vi "CheckPressure.vi"(8 "error in (no error)":errorcluster, 11 "UI.lvclass":refnum<class "S3.lvclass">) -> (0 "error out":errorcluster, 3 "UI.lvclass 2":refnum<class "S3.lvclass">)   [LabVIEW 2018, in "S3.lvclass"]
uses:
  S3.lvclass
  S3.lvclass/S3.ctl
  Public Controls/ReportHeader.ctl
  GUI2/GUI2.lvclass
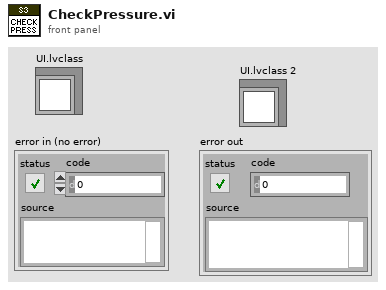
[diagram p1: front panel]
types:
  T1 = typedef "S3.lvclass/ReportHeader.ctl" = string
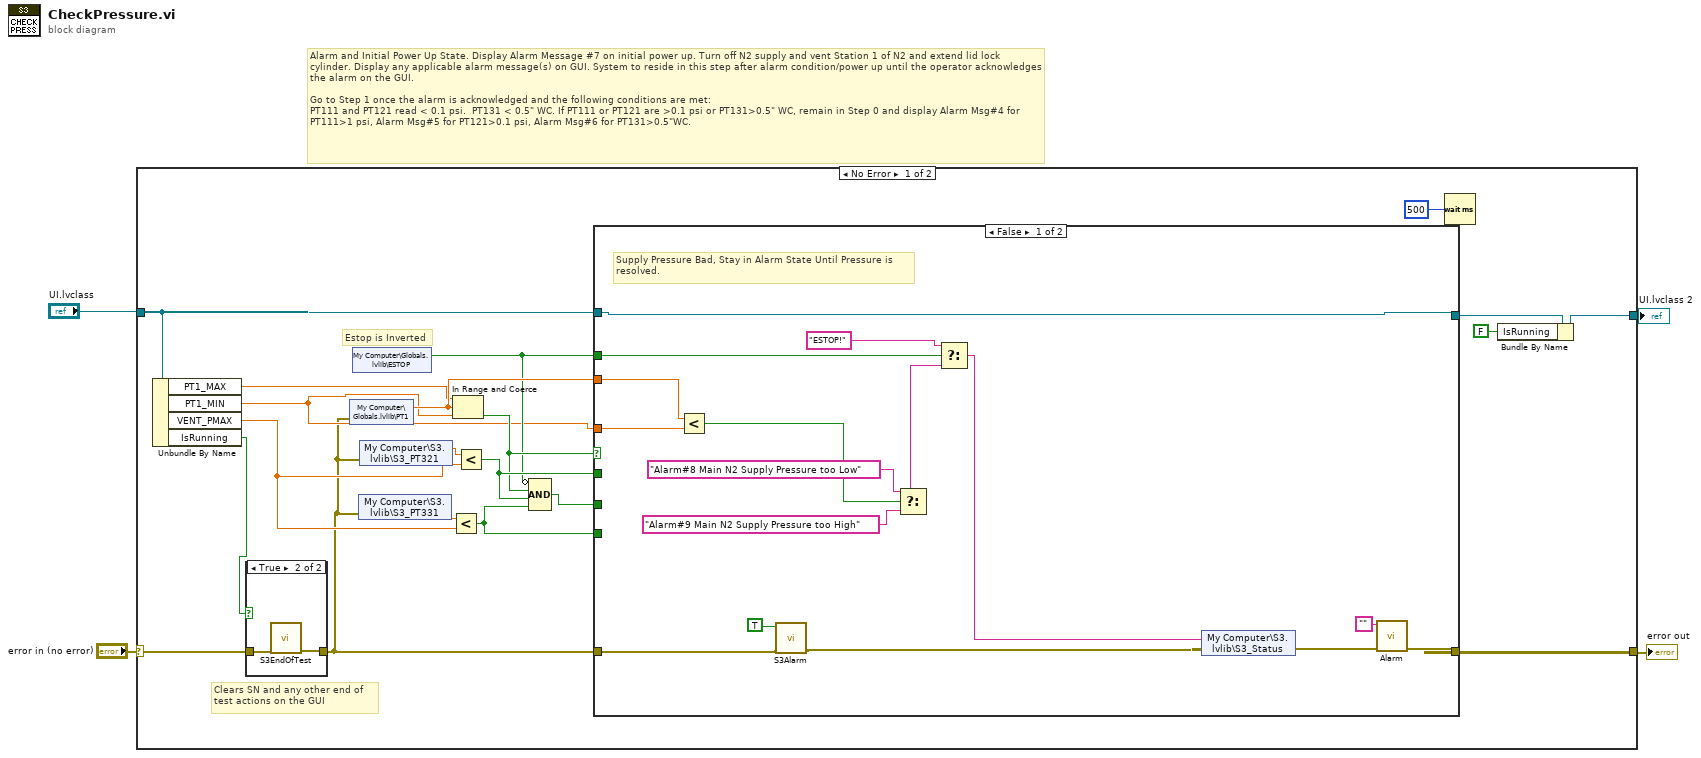
[diagram p0: block diagram]
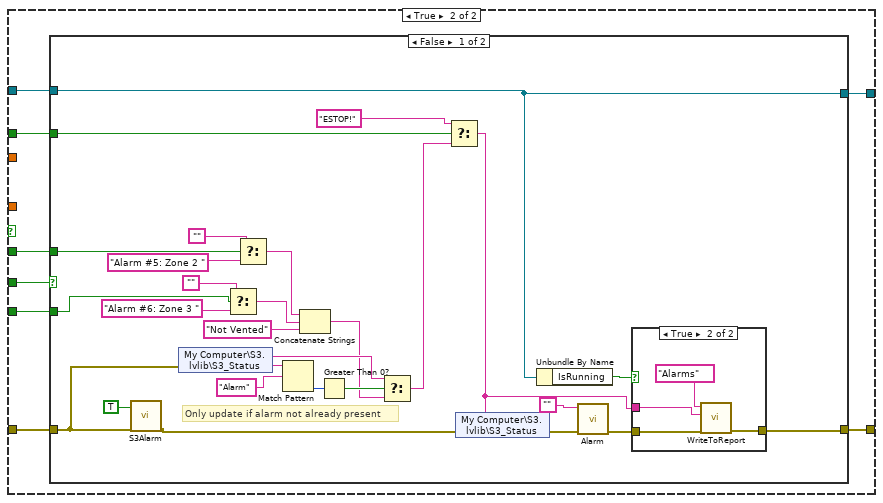
[diagram p3: hidden frame]
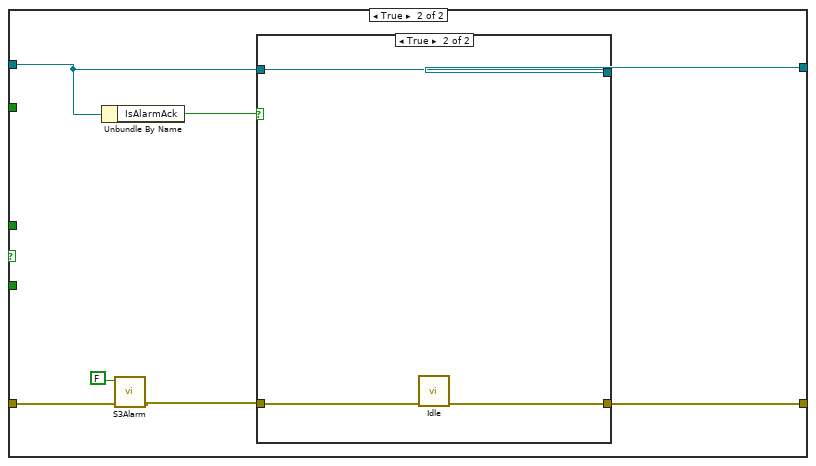
[diagram p5: hidden frame]
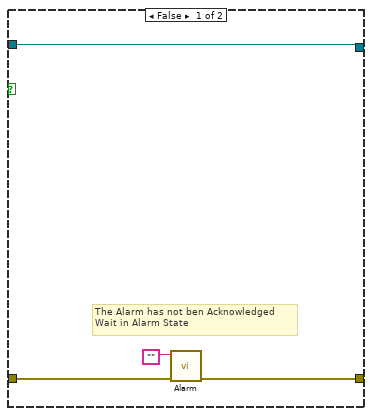
[diagram p6: hidden frame]
diagram:
  # "Alarm and Initial Power Up State. Display Alarm Message #7 on initial power up. Turn off N2 supply and vent Station 1 of N2 and extend lid lock cylinder. Display any applicable alarm message(s) on GUI. System to reside in this step after alarm condition/power up until the operator acknowledges the alarm on the GUI. \n\nGo to Step 1 once the alarm is acknowledged and the following conditions are met:\nPT111 and PT121 read < 0.1 psi.  PT131 < 0.5\" WC. If PT111 or PT121 are >0.1 psi or PT131>0.5\" WC, remain in Step 0 and display Alarm Msg#4 for PT111>1 psi, Alarm Msg#5 for PT121>0.1 psi, Alarm Msg#6 for PT131>0.5\"WC."
  n1 = case shown="No Error" "error in (no error)" {
    selector: "error in (no error)" -> [w8 w99]
    tunnel: [w21 w99] -> w3
    tunnel: "UI.lvclass" -> [w13 w98]
    tunnel: [w6 w98] -> w1
    frame No Error {
      # "Clears SN and any other end of\ntest actions on the GUI"
      # "Estop is Inverted"
      n2 = Unbundle By Name(w13) -> ("PT1_MAX"=w12:dbl, "PT1_MIN"=w11:dbl, "VENT_PMAX"=w10:dbl, "IsRunning"=w9:bool)
      n3 = case shown="True" w9 {
        tunnel: w8 -> [w25 w27]
        tunnel: [w25 w26] -> w7
        frame False {
        }
        frame True {
          n4 = call "S3EndOfTest.vi"("error in"=w27) -> ("error out"=w26:errorcluster)  [unwired: 10 in]
        }
      }
      n5 = shared-variable "My Computer\\Globals.lvlib\\PT1"(error in=w7) -> (w17:dbl)  [unwired: 1 out]
      n6 = shared-variable "My Computer\\Globals.lvlib\\ESTOP"() -> (w15:bool)  [unwired: 1 in, 1 out]
      n7 = shared-variable "My Computer\\S3.lvlib\\S3_PT331"(error in=w7) -> (w23:dbl)  [unwired: 1 out]
      n8 = shared-variable "My Computer\\S3.lvlib\\S3_PT321"(error in=w7) -> (w24:dbl)  [unwired: 1 out]
      n9 = Less?(x=w23, y=w10) -> (x < y?=w19:bool)
      n10 = In Range and Coerce(upper limit=w12, x=w17, lower limit=w11) -> (In Range?=w18:bool)  [unwired: 1 out]
      n11 = Less?(x=w24, y=w10) -> (x < y?=w20:bool)
      n12 = Compound Arithmetic op=AND(invert w15, w18, w20, w19) -> (w22:bool)
      n13 = case shown="False" w18 {
        tunnel: w22 -> [_ w51]
        tunnel: [w39 w50] -> w21
        tunnel: w20 -> [_ w49]
        tunnel: w19 -> [_ w48]
        tunnel: w7 -> [w29 w47]
        tunnel: w17 -> [w43 _]
        tunnel: w11 -> [w37 _]
        tunnel: w15 -> [w34 w46]
        tunnel: w13 -> [w36 w45]
        tunnel: [w36 w44] -> w14
        frame False {
          # "Supply Pressure Bad, Stay in Alarm State Until Pressure is\nresolved."
          n14 = Less?(x=w43, y=w37) -> (x < y?=w42:bool)
          n15 = call "S3Alarm.vi"("error in"=w29, "HasAlarm"=TRUE) -> ("error out"=w28:errorcluster)  [unwired: 9 in]
          n16 = Select(t="Alarm#8 Main N2 Supply Pressure too Low" ("Status"), s=w42, f="Alarm#9 Main N2 Supply Pressure too High" ("Status")) -> (s? t:f=w33:string)
          n17 = Select(t="ESTOP!" ("f"), s=w34, f=w33) -> (s? t:f=w32:string)
          n18 = shared-variable "My Computer\\S3.lvlib\\S3_Status"(w32, error in=w28) -> (error out=w40:errorcluster)
          n19 = call "Alarm.vi"("error in"=w40, "Alarm"="") -> ("error out"=w39:errorcluster)  [unwired: 9 in]
        }
        frame True {
          n20 = case shown="False" w51 {
            tunnel: w47 -> [w54 w85]
            tunnel: [w67 w90] -> w50
            tunnel: w49 -> [w77 _]
            tunnel: w48 -> [w72 _]
            tunnel: w46 -> [w65 _]
            tunnel: w45 -> [w63 w88]
            tunnel: [w63 w87] -> w44
            frame False {
              # "Only update if alarm not already present"
              n21 = call "S3Alarm.vi"("error in"=w54, "HasAlarm"=TRUE) -> ("error out"=w52:errorcluster)  [unwired: 9 in]
              n22 = shared-variable "My Computer\\S3.lvlib\\S3_Status"(error in=w54) -> (w59:string)  [unwired: 1 out]
              n23 = Select(t="", s=w72, f="Alarm #6: Zone 3 " ("Status")) -> (s? t:f=w70:string)
              n24 = Select(t="", s=w77, f="Alarm #5: Zone 2 " ("Status")) -> (s? t:f=w71:string)
              n25 = Match Pattern(string=w59, regular expression="Alarm") -> (offset past match=w61:i32)  [unwired: 1 in, 3 out]
              n26 = Concatenate Strings(w71, w70, "Not Vented" ("string")) -> (w58:string)
              n27 = Greater Than 0?(x=w61) -> (x > 0?=w60:bool)
              n28 = Select(t=w59, s=w60, f=w58) -> (s? t:f=w57:string)
              n29 = Select(t="ESTOP!" ("f"), s=w65, f=w57) -> (s? t:f=w56:string)
              n30 = shared-variable "My Computer\\S3.lvlib\\S3_Status"(w56, error in=w52) -> (error out=w78:errorcluster)
              n31 = Unbundle By Name(w63) -> ("IsRunning"=w64:bool)
              n32 = call "Alarm.vi"("error in"=w78, "Alarm"="") -> ("error out"=w68:errorcluster)  [unwired: 9 in]
              n33 = case shown="True" w64 {
                tunnel: w68 -> [w79 w83]
                tunnel: [w79 w82] -> w67
                tunnel: w56 -> [_ w80]
                frame False {
                }
                frame True {
                  n34 = call "WriteToReport.vi"("error in"=w83, "Value"=w80, "Header"=T1 "Alarms") -> ("error out"=w82:errorcluster)  [unwired: 8 in]
                }
              }
            }
            frame True {
              n35 = Unbundle By Name(w88) -> ("IsAlarmAck"=w89:bool)
              n36 = call "S3Alarm.vi"("error in"=w85, "HasAlarm"=FALSE) -> ("error out"=w84:errorcluster)  [unwired: 9 in]
              n37 = case shown="True" w89 {
                tunnel: w84 -> [w94 w97]
                tunnel: [w93 w96] -> w90
                tunnel: w88 -> [w92 w95]
                tunnel: [w92 w95] -> w87
                frame False {
                  # "The Alarm has not ben Acknowledged\nWait in Alarm State"
                  n38 = call "Alarm.vi"("error in"=w94, "Alarm"="") -> ("error out"=w93:errorcluster)  [unwired: 9 in]
                }
                frame True {
                  n39 = call "Idle.vi"("error in"=w97) -> ("error out"=w96:errorcluster)  [unwired: 10 in]
                }
              }
            }
          }
        }
      }
      n40 = Wait (ms)(milliseconds to wait=u32 500) -> ()  [unwired: 1 out]
      n41 = Bundle By Name(cluster=w14, "IsRunning"=FALSE) -> (w6:refnum<class "S3.lvclass">)
    }
    frame Error {
    }
  }
  "error out" <- w3
  "UI.lvclass 2" <- w1
